vi "eraseXY_img.vi"   [LabVIEW 2013]
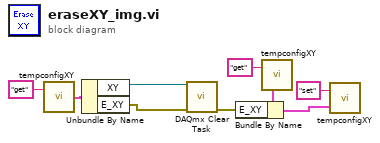
[diagram p0: block diagram]
diagram:
  n1 = call "tempconfigXY.vi"("command"="get") -> ("Temp Config out"=w4:cluster{" XY":refnum<k21>, "E_XY":errorcluster})  [unwired: 1 in]
  n2 = Unbundle By Name(w4) -> ("XY"=w2:refnum<k21>, "E_XY"=w1:errorcluster)
  n3 = call <vilib>:"DAQmx Clear Task.vi"("task in"=w2, "error in"=w1) -> ("error out"=w8:errorcluster)  [unwired: 13 in]
  n4 = call "tempconfigXY.vi"("command"="get") -> ("Temp Config out"=w7:cluster{" XY":refnum<k21>, "E_XY":errorcluster})  [unwired: 1 in]
  n5 = Bundle By Name(cluster=w7, "E_XY"=w8) -> (w9:cluster{" XY":refnum<k21>, "E_XY":errorcluster})
  n6 = call "tempconfigXY.vi"("Temp Config in"=w9, "command"="set") -> ()  [unwired: 1 out]
